vi "Flush Data Queuevi.vi"(8 "error in (no error)":errorcluster, 11 "DAQ Class in":refnum<class "DAQ Class.lvclass">) -> (0 "error out":errorcluster, 3 "DAQ Class out":refnum<class "DAQ Class.lvclass">)   [LabVIEW 2015, in "DAQ Class.lvclass"]
uses:
  DAQ Class.lvclass
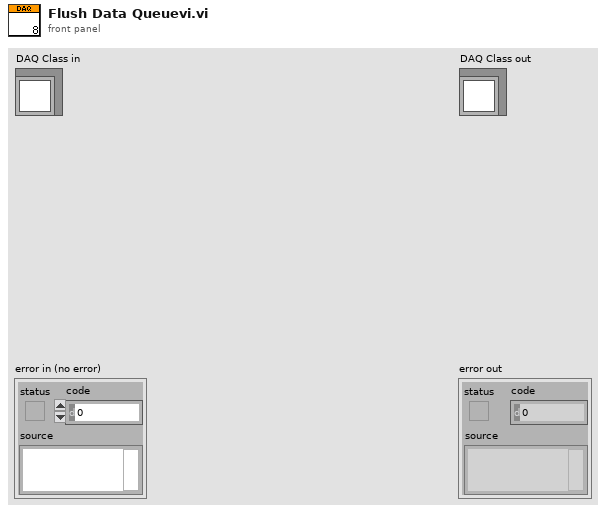
[diagram p1: front panel]
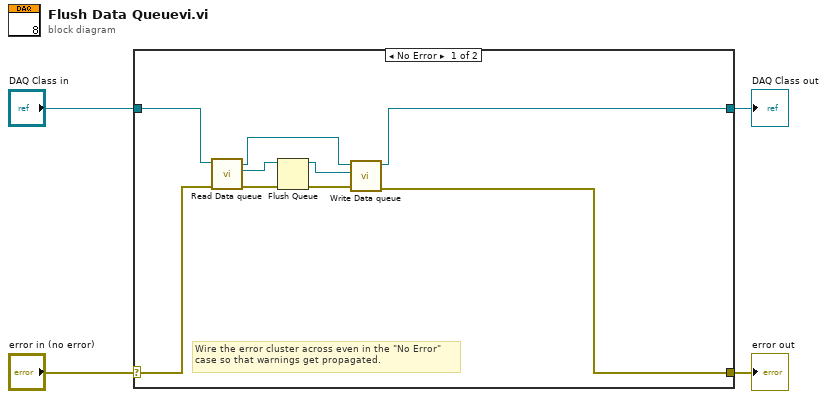
[diagram p0: block diagram]
diagram:
  n1 = case shown="No Error" "error in (no error)" {
    selector: "error in (no error)" -> [w11 w15]
    tunnel: [w7 w15] -> w3
    tunnel: [w6 w14] -> w1
    tunnel: "DAQ Class in" -> [w13 w14]
    frame No Error {
      # "Wire the error cluster across even in the \"No Error\"\ncase so that warnings get propagated."
      n2 = call-dynamic "Read Data queue.vi"("error in (no error)"=w11, "DAQ Class in"=w13) -> ("error out"=w8:errorcluster, "Data queue"=w12:refnum<queue>, "DAQ Class out"=w5:refnum<class "DAQ Class.lvclass">)  [unwired: 7 in]
      n3 = Flush Queue(queue=w12, error in (no error)=w8) -> (queue out=w9:refnum<queue>, error out=w10:errorcluster)  [unwired: 1 out]
      n4 = call-dynamic "Write Data queue.vi"("error in (no error)"=w10, "Data queue"=w9, "DAQ Class in"=w5) -> ("error out"=w7:errorcluster, "DAQ Class out"=w6:refnum<class "DAQ Class.lvclass">)  [unwired: 7 in]
    }
    frame Error {
    }
  }
  "error out" <- w3
  "DAQ Class out" <- w1
